vi "Stop Core.vi"(10 "final error code":i32, 11 "Logger in":refnum<class "Generic Logger.lvclass">) -> (3 "Logger out":refnum<class "Generic Logger.lvclass">)   [LabVIEW 2020, in "Logging.lvlib" / "Generic Logger.lvclass"]
doc: "(<B>Filename</B>: Actor Framework.lvlib:Actor.lvclass:Stop Core.vi)\n\nDefines what the actor does before it stops. Use the <B>final error code</B> input to determine whether the actor shut down in response to an error.\n\nBy default, this method passes the Stop message along to all auto-stop nested actors. A descendant class may override this method to define additional behavior, such as shutting down any processes the actor initiated in its override of the Actor Core method."
uses:
  Generic Logger.lvclass
  Generic Logger.lvclass/Generic Logger.ctl
  <vilib>/ActorFramework/Actor/Actor.lvclass
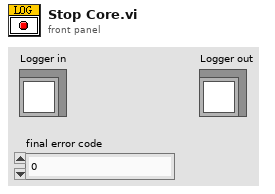
[diagram p1: front panel]
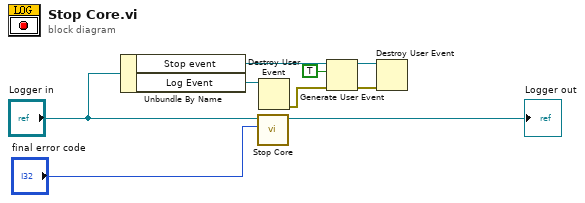
[diagram p0: block diagram]
diagram:
  n1 = Unbundle By Name("Logger in") -> ("Stop event"=w6:refnum<user-event>, "Log Event"=w7:refnum<user-event>)
  n2 = call-parent "Stop Core.vi"("final error code"="final error code", "Actor in"="Logger in") -> ("Actor out"=→"Logger out":refnum<class "Generic Logger.lvclass">)  [unwired: 9 in]
  n3 = Destroy User Event(user event=w7) -> (error out=w3:errorcluster)  [unwired: 1 in]
  n4 = Generate User Event(user event=w6, event data cluster=TRUE ("event data"), error in=w3) -> (user event out=w5:refnum<user-event>, error out=w2:errorcluster)  [unwired: 1 in]
  n5 = Destroy User Event(user event=w5, error in=w2) -> ()  [unwired: 1 out]
